vi "Read Splitter Refnum.vi"(8 "error in (no error)":errorcluster, 11 "Docking in":refnum<class "Docking.lvclass">) -> (0 "error out":errorcluster, 2 "Splitter Refnum":refnum<vi>, 3 "Docking out":refnum<class "Docking.lvclass">)   [LabVIEW 2023, in "Docking.lvlib" / "Docking.lvclass"]
doc: "Returns a refnum to the splitter that is adjusted to show/hide the docked actor."
uses:
  Docking.lvclass
  Docking.lvclass/Docking.ctl
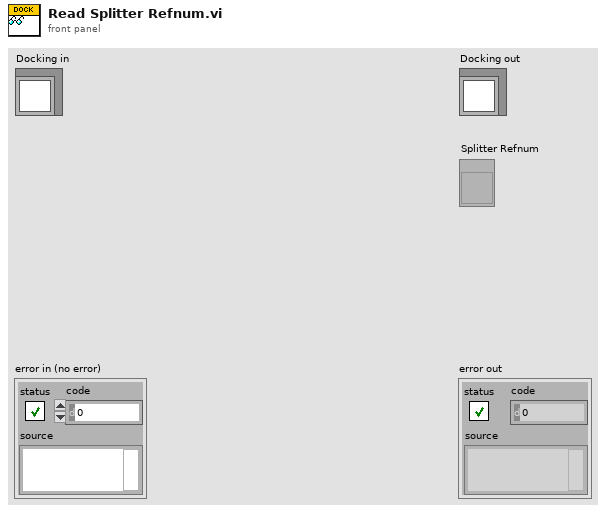
[diagram p1: front panel]
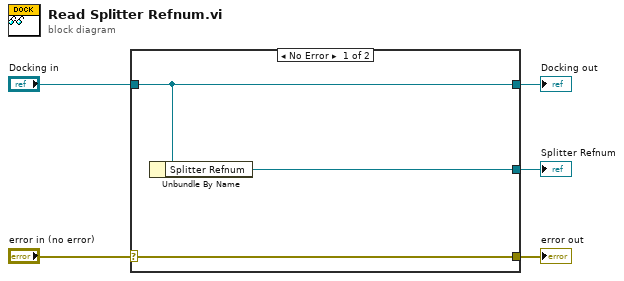
[diagram p0: block diagram]
diagram:
  n1 = case shown="No Error" "error in (no error)" {
    selector: "error in (no error)" -> [w8 w9]
    tunnel: [w8 w9] -> w4
    tunnel: [w7 w10] -> w2
    tunnel: "Docking in" -> [w7 w10]
    tunnel: [w6 _] -> w1
    frame No Error {
      n2 = Unbundle By Name(w7) -> ("Splitter Refnum"=w6:refnum<vi>)
    }
    frame Error {
    }
  }
  "error out" <- w4
  "Docking out" <- w2
  "Splitter Refnum" <- w1
